vi "Limelight Set Pipeline.vi"(8 "error in (no error)":errorcluster, 11 "Pipeline number":i8=9) -> (0 "error out":errorcluster)   [LabVIEW 2019]
uses:
  <vilib>/Rock Robotics/Network Tables/NT Write Number.vi
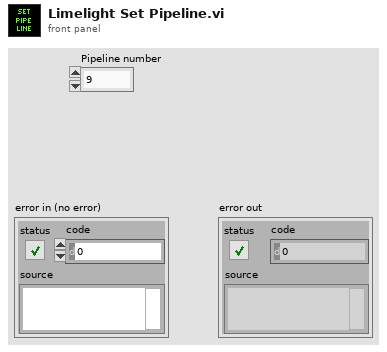
[diagram p1: front panel]
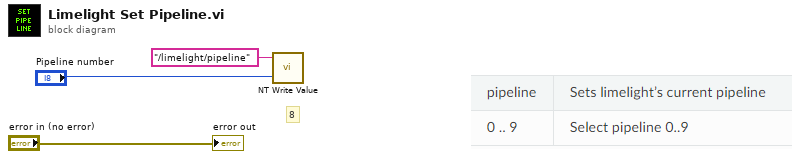
[diagram p0: block diagram]
diagram:
  # "8"
  n1 = call-poly <vilib>:"NT Write Value.vi"("Numeric"="Pipeline number", "Name"="/limelight/pipeline") -> ()  [unwired: 9 in, 1 out]
  "error out" <- "error in (no error)"
